vi "Numeric Alarm.vi"(10 "Simple Alarm Values":T1={"tag name"="mytag", "HiHi"=90.0, "Hi"=75.0, "Lo"=25.0, "LoLo"=10.0, "alarm delay"=0.0}, 11 "Alarms in":T2[](array[typedef])) -> (3 "Alarms out":T2[](array[typedef]))   [LabVIEW 2018, in "Dynamic Shared Variables.lvlib"]
doc: "Create a numeric alarm configuration with some defaults."
uses:
  Dynamic Shared Variables.lvlib
  Tag VIs/Numeric Alarm Settings Cluster.ctl
  Simple Alarm Values Cluster.ctl
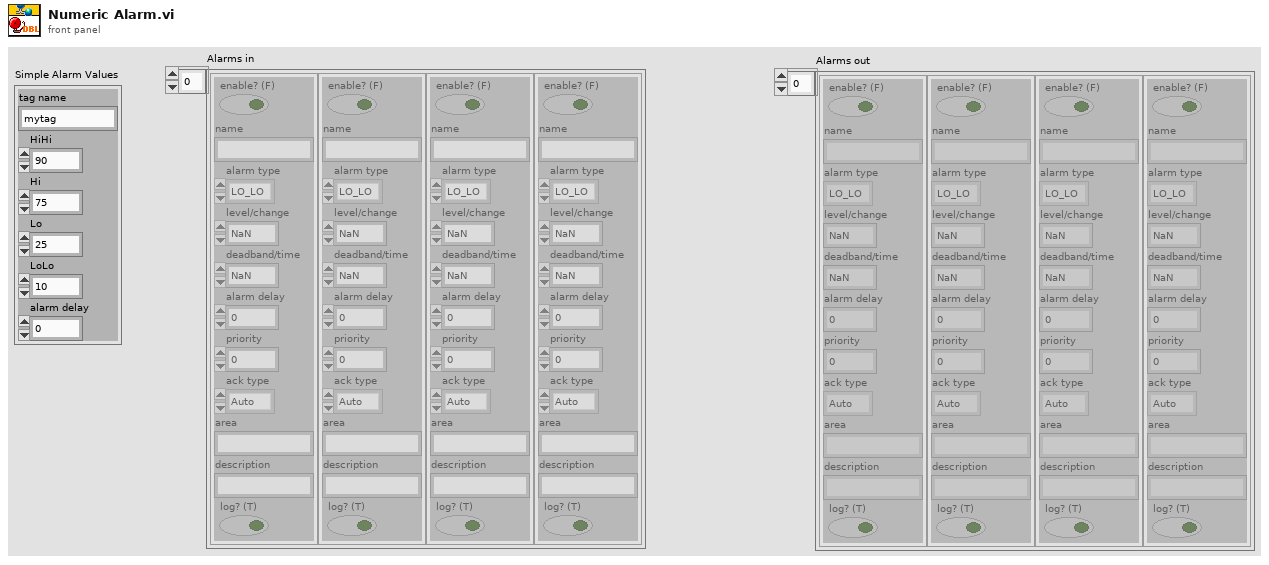
[diagram p1: front panel]
types:
  T1 = typedef "Dynamic Shared Variables.lvlib/Simple Alarm Values Cluster.ctl" = cluster{"tag name":string, "HiHi":dbl, "Hi":dbl, "Lo":dbl, "LoLo":dbl, "alarm delay":dbl}
  T2 = typedef "Numeric Alarm Settings Cluster.ctl" = cluster{"enable? (F)":bool, "name":string, "alarm type":enum16{"HI_HI", "HI", "LO", "LO_LO"}, "level/change":dbl, "deadband/time":dbl, "alarm delay":dbl, "priority":u32, "ack type":enum16{"Auto", "User", "None", "Each Occurrence"}, "area":string, "description":string, "log? (T)":bool}
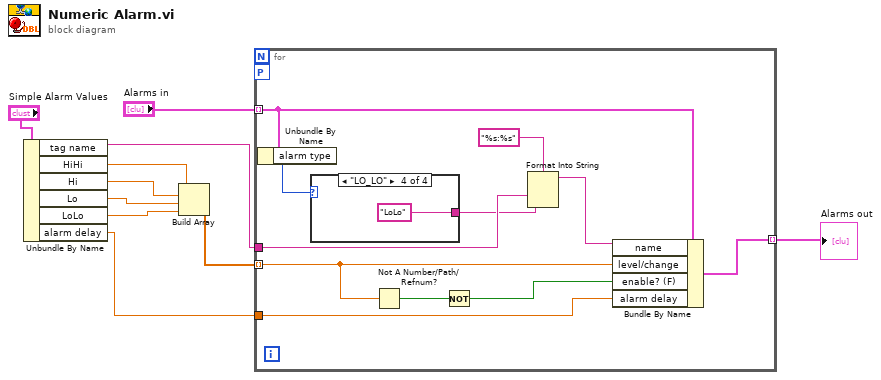
[diagram p0: block diagram]
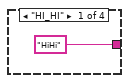
[diagram p2: hidden frame]
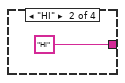
[diagram p3: hidden frame]
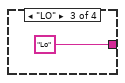
[diagram p4: hidden frame]
diagram:
  n1 = Unbundle By Name("Simple Alarm Values") -> ("tag name"=w6:string, "HiHi"=w5:dbl, "Hi"=w4:dbl, "Lo"=w3:dbl, "LoLo"=w2:dbl, "alarm delay"=w1:dbl)
  n2 = Build Array(w5, w4, w3, w2) -> (w9:dbl[])
  n3 = for {
    tunnel: w6 -> [w17]
    tunnel: "Alarms in" -> [w20] mode=indexing
    tunnel: w9 -> [w14] mode=indexing
    tunnel: [w21] -> w8 mode=indexing
    tunnel: w1 -> [w11]
    workers-P: _ -> [_]
    n4 = Unbundle By Name(w20) -> ("alarm type"=w19:enum16{"HI_HI", "HI", "LO", "LO_LO"})
    n5 = case shown="\"LO_LO\"" w19 {
      tunnel: ["HiHi" "Hi" "Lo" "LoLo"] -> w16
      frame "HI_HI" {
      }
      frame "HI" {
      }
      frame "LO" {
      }
      frame "LO_LO" {
      }
    }
    n6 = Not A Number/Path/Refnum?(number/path/refnum=w14) -> (NaN/Path/Refnum?=w13:bool)
    n7 = Not(x=w13) -> (.not. x?=w12:bool)
    n8 = Format Into String(format string="%s:%s", w17, w16) -> (resulting string=w15:string)  [unwired: 2 in, 1 out]
    n9 = Bundle By Name(cluster=w20, "name"=w15, "level/change"=w14, "enable? (F)"=w12, "alarm delay"=w11) -> (w21:T2)
  }
  "Alarms out" <- w8
